vi "DecimalToBinary.vi"(1 "Resolution":i32=13, 2 "Decimal":dbl) -> (0 "Binary":bool[](array[boolean]))   [LabVIEW 2013]
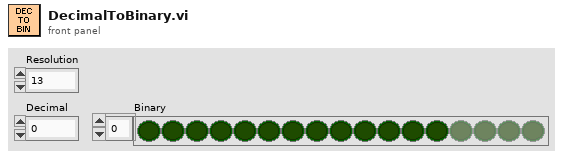
[diagram p1: front panel]
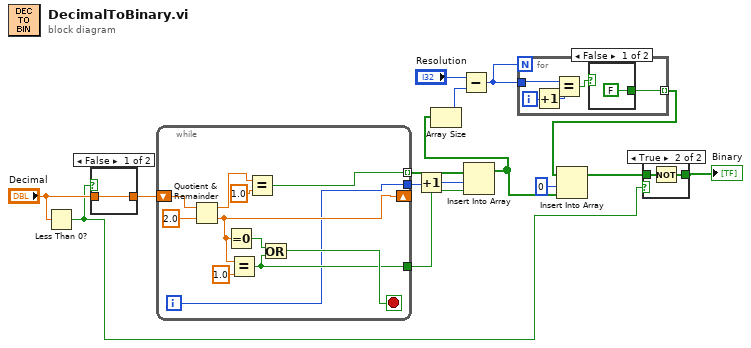
[diagram p0: block diagram]
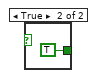
[diagram p2: hidden frame]
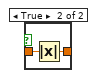
[diagram p4: hidden frame]
diagram:
  n1 = Less Than 0?(x="Decimal") -> (x < 0?=w10:bool)
  n2 = case shown="False" w10 {
    tunnel: "Decimal" -> [w16 w18]
    tunnel: [w16 w17] -> w12
    frame False {
    }
    frame True {
      n3 = Absolute Value(x=w18) -> (abs(x)=w17:dbl)
    }
  }
  n4 = while {
    shift-right: [w23] -> _
    shift-left: w12 -> [w29]
    tunnel: [w21] -> w6 mode=indexing
    tunnel: [w20] -> w15
    tunnel: [w19] -> w14
    i -> [w19]
    stop <- w22 stop-if-true
    n5 = Quotient & Remainder(x=w29, y=2.0) -> (x-y*floor(x/y)=w27:dbl, floor(x/y)=w23:dbl)
    n6 = Equal To 0?(x=w23) -> (x = 0?=w25:bool)
    n7 = Equal?(x=w23, y=1.0) -> (x = y?=w20:bool)
    n8 = Equal?(x=w27, y=1.0) -> (x = y?=w21:bool)
    n9 = Or(x=w25, y=w20) -> (x .or. y?=w22:bool)
  }
  n10 = Increment(x=w14) -> (x+1=w11:i32)
  n11 = Insert Into Array(array=w6, index=w11, new element=w15) -> (w2:bool[])
  n12 = Array Size(array=w2) -> (size(s)=w5:i32)
  n13 = Subtract(x="Resolution", y=w5) -> (x-y=w4:i32)
  n14 = for {
    N: w4 -> [_]
    tunnel: w4 -> [w31]
    tunnel: [w30] -> w3 mode=indexing
    i -> [w34]
    n15 = Increment(x=w34) -> (x+1=w32:i32)
    n16 = Equal?(x=w31, y=w32) -> (x = y?=w33:bool)
    n17 = case shown="False" w33 {
      tunnel: [FALSE TRUE] -> w30
      frame False {
      }
      frame True {
      }
    }
  }
  n18 = Insert Into Array(array=w3, index=0, new element=w2) -> (w9:bool[])
  n19 = case shown="True" w10 {
    tunnel: w9 -> [w37 w39]
    tunnel: [w37 w38] -> w8
    frame False {
    }
    frame True {
      n20 = Not(x=w39) -> (.not. x?=w38:bool[])
    }
  }
  "Binary" <- w8
